vi "Read All Information.vi"() -> ()   [LabVIEW 2020]
uses:
  <vilib>/addons/database/NI_Database_API.lvlib
panel:
  in  "error in (no error)":errorcluster
  out "Database Information":string[][](table)
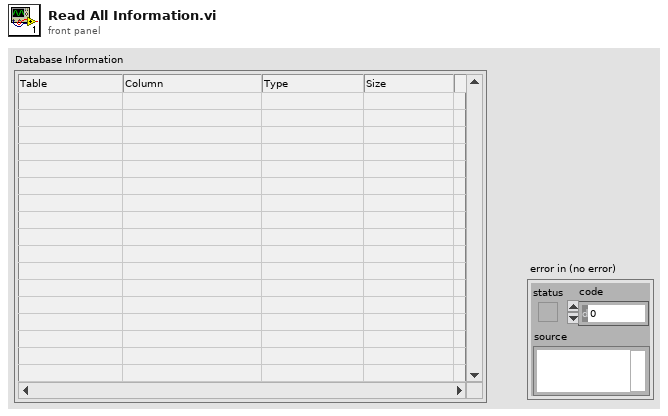
[diagram p1: front panel]
types:
  T1 = typedef "NI_Database_API.lvlib/Conn ObjectReference.ctl" = refnum<k1>
  T2 = typedef "NI_Database_API.lvlib/DB Tools DataTypes.ctl" = enum16{"String", "Long (I32)", "Single (SGL)", "Double (DBL)", "Date/Time", "Binary"}
  T3 = cluster{"name":string, "database data type":T2, "defined size":i32}[]
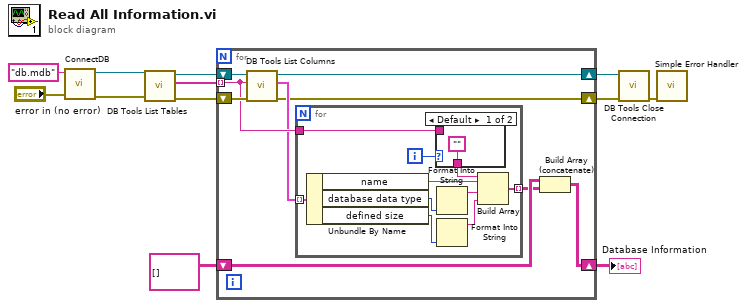
[diagram p0: block diagram]
diagram:
  n1 = call "ConnectDB.vi"("error in (no error)"="error in (no error)", "Filename"="db.mdb") -> ("error out"=w1:errorcluster, "DB Conn"=w2:T1)  [unwired: 8 in]
  n2 = call <vilib>:"DB Tools List Tables.vi"("error in (no error)"=w1, "connection reference"=w2) -> ("error out"=w11:errorcluster, "tables"=w10:string[], "connection reference out"=w12:T1)  [unwired: 3 in]
  n3 = for {
    shift-right: [w17] -> w7
    shift-left: w11 -> [w21]
    tunnel: w10 -> [w19] mode=indexing
    shift-right: [w16] -> w9
    shift-left: string[][] [] -> [w15]
    shift-right: [w13] -> w6
    shift-left: w12 -> [w20]
    n4 = call <vilib>:"DB Tools List Columns.vi"("error in (no error)"=w21, "table"=w19, "connection reference"=w20) -> ("error out"=w17:errorcluster, "column information"=w18:T3, "connection reference out"=w13:T1)  [unwired: 1 in, 1 out]
    n5 = for {
      tunnel: w19 -> [w30]
      tunnel: w18 -> [w27] mode=indexing
      tunnel: [w29] -> w14 mode=indexing
      i -> [w31]
      n6 = Unbundle By Name(w27) -> ("name"=w26:string, "database data type"=w25:T2, "defined size"=w23:i32)
      n7 = case shown="Default" w31 {
        tunnel: w30 -> [_ w33]
        tunnel: ["" w33] -> w28
        frame Default {
        }
        frame 0 {
        }
      }
      n8 = Format Into String(w25) -> (resulting string=w24:string)  [unwired: 3 in, 1 out]
      n9 = Format Into String(w23) -> (resulting string=w22:string)  [unwired: 3 in, 1 out]
      n10 = Build Array(w28, w26, w24, w22) -> (w29:string[])
    }
    n11 = Build Array (concatenate)(w15, w14) -> (w16:string[][])
  }
  "Database Information" <- w9
  n12 = call <vilib>:"DB Tools Close Connection.vi"("error in (no error)"=w7, "connection reference"=w6) -> ("error out"=w5:errorcluster)  [unwired: 5 in]
  n13 = call <vilib>:"Simple Error Handler.vi"("error in (no error)"=w5) -> ()  [unwired: 4 in, 5 out]
